vi "Pretty Print.vi"(4 "Disable LabVIEW Extensions":bool, 7 "Comment out unparsable lines":bool, 8 "error in (no error)":errorcluster, 10 "Offset":i32, 11 "JSON":string) -> (0 "error out":errorcluster, 2 "Rest of Input String":string, 3 "<JSON>":string caption="<JSON>First JSON Value")   [LabVIEW 2020, in "JSONtext.lvlib"]
doc: "\"Pretty print\" with extra whitespace and new lines to make the JSON more human readable.\n\nThis method uses a different algorithm from the \"Reformat\" method. Differences\n-- faster\n-- supports comments\n-- does not serve to verify the correctness of the input JSON, like Reformat does."
uses:
  <vilib>/JDP Science/JSONtext/JSONtext.lvlib
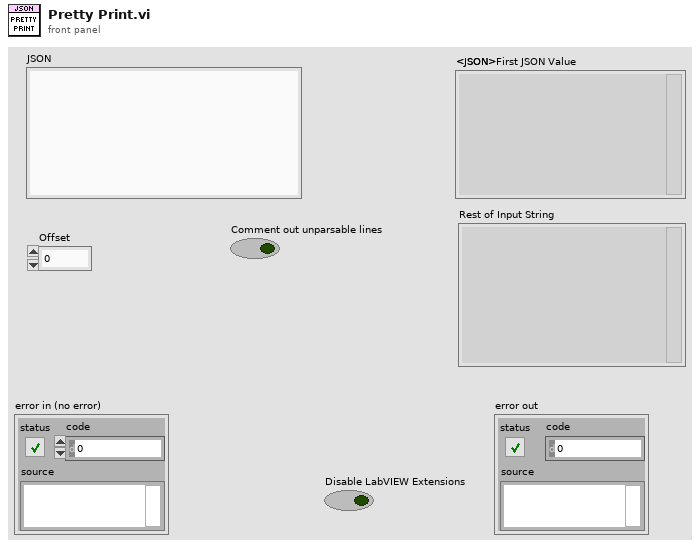
[diagram p1: front panel]
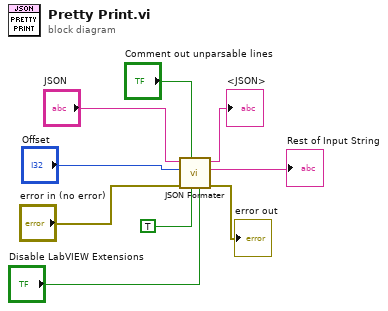
[diagram p0: block diagram]
diagram:
  n1 = call <vilib>:"JSON Formater.vi"("Disable LabVIEW Extensions"="Disable LabVIEW Extensions", "Pretty Print"=TRUE, "Comment out unparsable lines"="Comment out unparsable lines", "error in"="error in (no error)", "Offset"="Offset", "JSON"="JSON") -> ("error OUT"=→"error out":errorcluster, "Rest of Input String"=→"Rest of Input String":string, "<JSON>"=→"<JSON>":string)  [unwired: 3 in]
